vi "Reset Auto Increment.vi"(8 "error in (no error)":errorcluster, 11 "VISA resource name":refnum<visa-resource-name>) -> (0 "error out":errorcluster, 3 "VISA resource name out":refnum<visa-resource-name>)   [LabVIEW 2018, in "EFD Ultimus V.lvlib"]
doc: "Resets the Auto Increment functions. The Ultimus V will set the Memory Address to the Start Address Value, reset the counters, and clear auto increment alarm. If the Ultimus V is not in counter or timer mode, the dispenser will return an error (A2). \n\nHost Format: SE--"
uses:
  EFD Ultimus V.lvlib
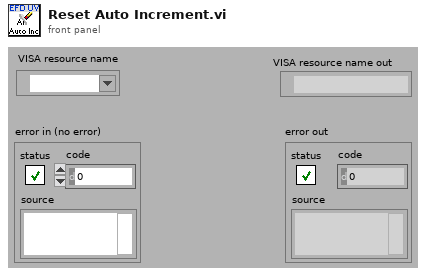
[diagram p1: front panel]
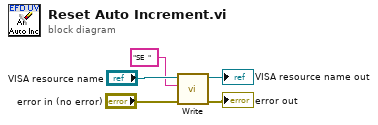
[diagram p0: block diagram]
diagram:
  n1 = call "Write.vi"("error in (no error)"="error in (no error)", "Command To Write"="SE  ", "VISA resource name"="VISA resource name") -> ("error out"=→"error out":errorcluster, "VISA resource name out"=→"VISA resource name out":refnum<visa-resource-name>)  [unwired: 7 in]
